vi "Speaker Change.vi"(8 "error in":errorcluster, 11 "cPAS in":refnum<class "cPAS.lvclass">) -> (0 "error out":errorcluster, 3 "cPAS out":refnum<class "cPAS.lvclass">)   [LabVIEW 2015, in "cPAS.lvclass"]
uses:
  cPAS.lvclass
  cPAS.lvclass/cPAS.ctl
  <vilib>/Utility/error.llb/Error Cluster From Error Code.vi
  <vilib>/rvi/errors/niLvFpgaAdjustHostInterfaceError.vi
  <vilib>/rvi/interface/nirviReadWriteControl/nirviReadWriteControl.xnode
  Interface/fpga_ctl.ctl
  FPGA Bitfiles/FPGA Server.lvbitx
  NiFpgaLv.dll
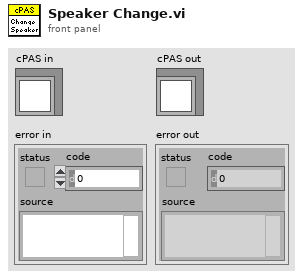
[diagram p1: front panel]
types:
  T1 = typedef "fpga_ctl.ctl" = refnum<k20>
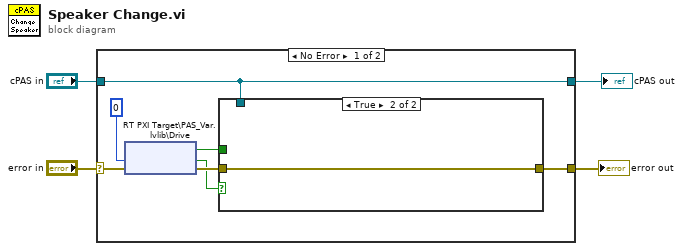
[diagram p0: block diagram]
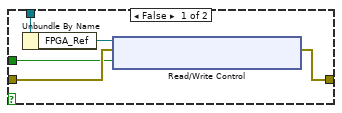
[diagram p2: hidden frame]
diagram:
  n1 = case shown="No Error" "error in" {
    selector: "error in" -> [w9 w19]
    tunnel: [w10 w19] -> w1
    tunnel: [w11 w18] -> w2
    tunnel: "cPAS in" -> [w11 w18]
    frame No Error {
      n2 = shared-variable "RT PXI Target\\PAS_Var.lvlib\\Drive"(error in=w9, 0 ("ms timeout (0)")) -> (w5:bool, error out=w7:errorcluster, w6:bool)
      n3 = case shown="True" w6 {
        tunnel: w11 -> [w16 _]
        tunnel: w7 -> [w14 w17]
        tunnel: [w13 w17] -> w10
        tunnel: w5 -> [w12 _]
        frame False {
          n4 = Unbundle By Name(w16) -> ("FPGA_Ref"=w15:T1)
          n5 = xnode "Read/Write Control"("FPGA VI Reference In"=w15, "error in"=w14, "Spk Enable"=w12) -> ("error out"=w13:errorcluster)  [unwired: 1 out]
        }
        frame True {
        }
      }
    }
    frame Error {
    }
  }
  "error out" <- w1
  "cPAS out" <- w2
